vi "updateAppNameAndVITitle.vi"() -> ()   [LabVIEW 2014]
uses:
  <vilib>/AppBuilder/AB_API_Simple/NI_App_Builder_API.lvlib
  <vilib>/AppBuilder/AB_API_Simple/Get Build Specification Version (path).vi
  <vilib>/AppBuilder/AB_API_Simple/Set Build Specification Version (path).vi
  <vilib>/AppBuilder/AB_API_Simple/Build (path).vi
  <vilib>/AppBuilder/AB_API_Simple/Build Specification Version.ctl
panel:
  out "Build Specification Version":T1
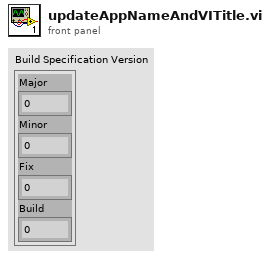
[diagram p1: front panel]
types:
  T1 = typedef "NI_App_Builder_API.lvlib/Build Specification Version.ctl" = cluster{"Major":u16, "Minor":u16, "Fix":u16, "Build":u16}
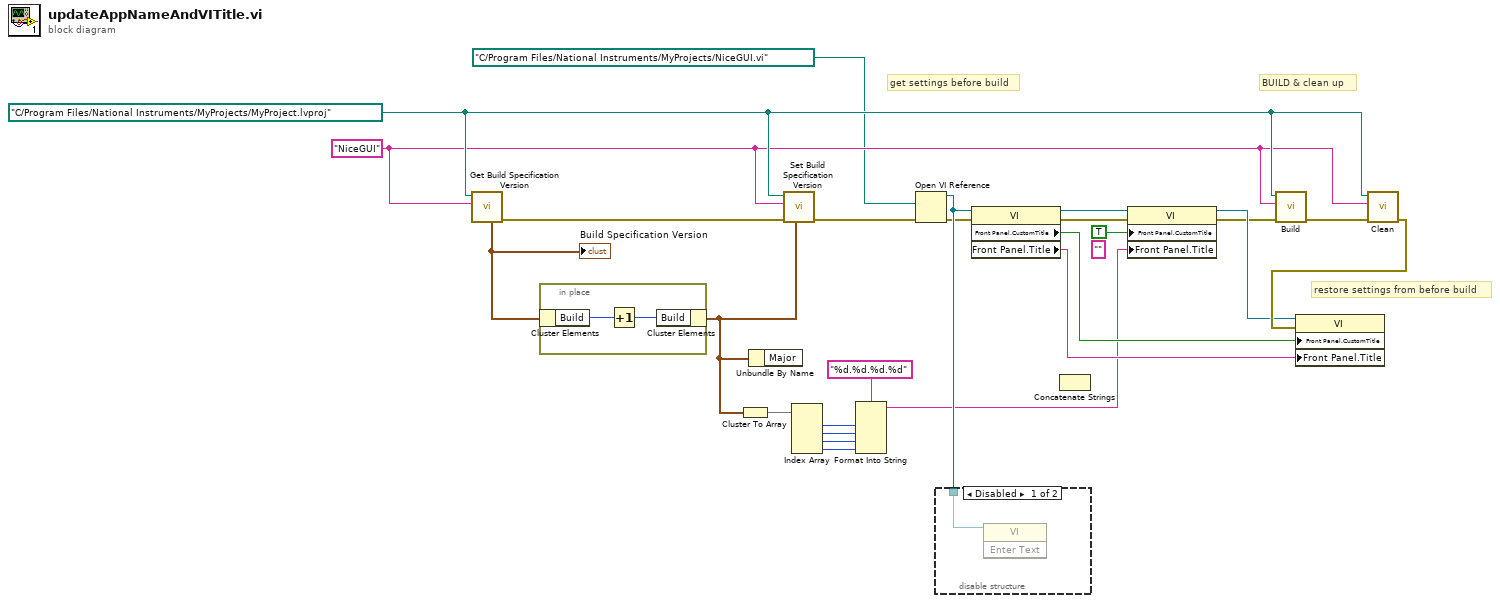
[diagram p0: block diagram]
diagram:
  (unwired) "" ("Front Panel Window:Title")
  w21 = "NiceGUI" ("Name of build specification")
  w22 = path "C:/Program Files/National Instruments/MyProjects/MyProject.lvproj" ("Path to project")
  # "restore settings from before build"
  # "BUILD & clean up"
  # "get settings before build"
  n1 = call-poly <vilib>:"Get Build Specification Version.vi"("Name of build specification"=w21, "Path to project"=w22) -> ("error out"=w25:errorcluster, "Build Specification Version"=w24:T1)  [unwired: 8 in]
  "Build Specification Version" <- w24
  n2 = in-place {
    n3 = in-place-cluster #1(w24) -> ("Build"=w27:u16)
    n4 = Increment(x=w27) -> (x+1=w26:u16)
    n5 = in-place-cluster #1("Build"=w26) -> (w8:T1)
  }
  n6 = Cluster To Array(cluster=w8) -> (array=w6:u16[])
  n7 = Unbundle By Name(w8) -> ()  [unwired: 1 out]
  n8 = call-poly <vilib>:"Set Build Specification Version.vi"("Build Specification Version"=w8, "error in (no error)"=w25, "Name of build specification"=w21, "Path to project"=w22) -> ("error out"=w19:errorcluster)  [unwired: 7 in]
  n9 = Index Array(array=w6) -> (element #1=w5:u16, element #2=w4:u16, element #3=w3:u16, element #4=w2:u16)  [unwired: 4 in]
  n10 = Format Into String(format string="%d.%d.%d.%d", w5, w4, w3, w2) -> (resulting string=w1:string)  [unwired: 2 in, 1 out]
  n11 = Open VI Reference(vi path=path "C:/Program Files/National Instruments/MyProjects/NiceGUI.vi", error in (no error)=w19) -> (vi reference=w18:refnum<vi>, error out=w17:errorcluster)  [unwired: 4 in]
  n12 = disable-structure shown="Disabled" {
    disable-tunnel: w18 -> [w28 _]
    frame Disabled {
      n13 = invoke class="VI" method="Enter Text"(reference=w28) -> ()  [unwired: 2 in, 3 out]
    }
    frame Enabled {
    }
  }
  n14 = property class="VI"(reference=w18, error in=w17) -> (reference out=w14:refnum<vi>, error out=w15:errorcluster, "Front Panel.CustomTitle"=w10:bool, "Front Panel.Title"=w11:string)
  n15 = Concatenate Strings() -> ()  [unwired: 2 in, 1 out]
  n16 = property class="VI"(reference=w14, error in=w15, "Front Panel.CustomTitle"=TRUE ("Front Panel Window:Custom Title"), "Front Panel.Title"=w1) -> (reference out=w13:refnum<vi>, error out=w12:errorcluster)
  n17 = call-poly <vilib>:"Build.vi"("error in (no error)"=w12, "Name of build specification (if empty: build all)"=w21, "Path to project"=w22) -> ("error out"=w23:errorcluster)  [unwired: 7 in, 1 out]
  n18 = call <vilib>:"Clean.vi"("error in (no error)"=w23, "Name of build specification (if empty: clean all)"=w21, "Path to project"=w22) -> ("error out"=w16:errorcluster)  [unwired: 8 in]
  n19 = property class="VI"(reference=w13, error in=w16, "Front Panel.CustomTitle"=w10, "Front Panel.Title"=w11) -> ()  [unwired: 2 out]
